vi "SetRemoteandTimeout.vi"(2 "error IO":errorcluster, 3 "VISA resource":refnum<visa-resource-name>) -> (0 "error":errorcluster, 1 "dup VISA resource":refnum<visa-resource-name>)   [LabVIEW 2020]
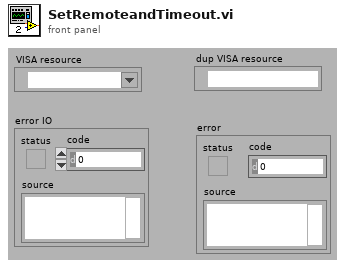
[diagram p1: front panel]
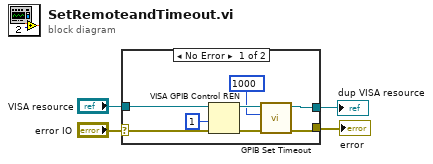
[diagram p0: block diagram]
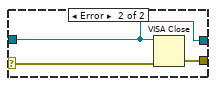
[diagram p2: hidden frame]
diagram:
  n1 = case shown="No Error" "error IO" {
    selector: "error IO" -> [w11 w14]
    tunnel: [w7 w15] -> w3
    tunnel: "VISA resource" -> [w12 w13]
    tunnel: [w6 w13] -> w2
    frame No Error {
      n2 = VISA GPIB Control REN(8:w11, 10:u16 1 ("mode"), 11:w12) -> (0:w10:errorcluster, 3:w9:refnum<visa-resource-name>)
      n3 = call "GPIB Set Timeout.vi"("Error In"=w10, "Timeout"=u32 1000, "VISA resource name"=w9) -> ("Error Out"=w7:errorcluster, "dup VISA resource name"=w6:refnum<visa-resource-name>)  [unwired: 2 in, 1 out]
    }
    frame Error {
      n4 = VISA Close(VISA resource name=w13, error in (no error)=w14) -> (error out=w15:errorcluster)
    }
  }
  "error" <- w3
  "dup VISA resource" <- w2
